vi "Untitled 5.vi"() -> ()   [LabVIEW 2015]
uses:
  <vilib>/NI_Real-Time Target Support.lvlib
panel:
  in  "stop":bool
  out "Total (%)":dbl(graph)
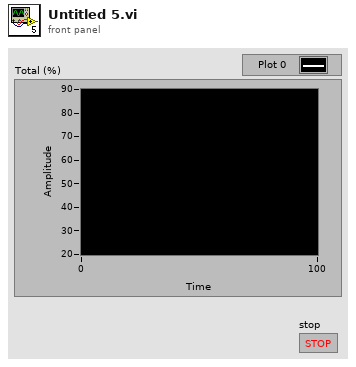
[diagram p1: front panel]
types:
  T1 = typedef "NI_Real-Time Target Support.lvlib/RT CPU Load.ctl" = cluster{"Total (%)":dbl, "Time Critical (%)":dbl, "Timed Structures (%)":dbl, "High (%)":dbl, "Above Normal (%)":dbl, "Normal (%)":dbl, "Background (%)":dbl, "Idle (%)":dbl, "ISR (%)":dbl}
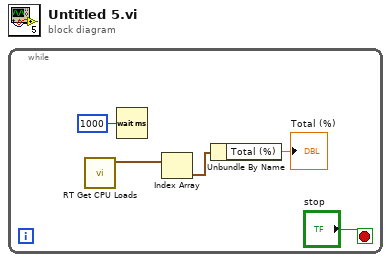
[diagram p0: block diagram]
diagram:
  n1 = while {
    stop <- "stop" stop-if-true
    n2 = call <vilib>:"RT Get CPU Loads.vi"() -> ("CPU loads"=w4:T1[])  [unwired: 10 in, 1 out]
    n3 = Wait (ms)(milliseconds to wait=u32 1000) -> ()  [unwired: 1 out]
    n4 = Index Array(array=w4) -> (element=w5:T1)  [unwired: 1 in]
    n5 = Unbundle By Name(w5) -> ("Total (%)"=→"Total (%)":dbl)
  }
